vi "MIDI_JamSession_run-me.vi"() -> ()   [LabVIEW 2013]
doc: "Render a standard MIDI file to a audio using user-defined subVIs as the \"instruments\" in \"The Band.\""
uses:
  Instance           1 30Saved   MIDI_JamSession_run-me .vi
  <vilib>/Analysis/NI_AALBase.lvlib
  Instance           2 30Saved   MIDI_JamSession_run-me .vi
  Instance           3 30Saved   MIDI_JamSession_run-me .vi
  <vilib>/Analysis/baseanly.llb/Quick Scale 2D.vi
  <vilib>/Utility/file.llb/Write To Spreadsheet File (DBL).vi
panel:
  out "playing audio":bool
  in  "lock pan":bool
  in  "lock mute":bool
  in  "lock preview":bool
  in  "lock instrument":bool
  in  "preview":bool[](array[boolean])=[TRUE, TRUE, TRUE, TRUE, TRUE, TRUE, TRUE, TRUE, TRUE, TRUE, TRUE, TRUE, TRUE, TRUE, TRUE, TRUE]
  in  "random pan":bool
  in  "note events output file (.csv)":path
  out "end":string="0:00"
  out "begin":string="0:00"
  out "duration":string="0:00"
  in  "About":bool
  in  "Show help":bool
  in  "Listen":bool=TRUE
  in  "Time range to render":cluster{i32, i32}(slide)={0, 10} scale=0.0..100.0
  in  "fs [Hz]":dbl=11025.0
  in  "pan (left <==> right)":i32[](array[slide])=[0, 0, 0, 0, 0, 0, 0, 0, 0, 0, 0, 0, 0, 0, 0, 0] min=-10 max=10 scale=-10.0..10.0
  out "Audio rendering progress":u8(slide) scale=0.0..100.0
  in  "mute":bool[](array[boolean])=[FALSE, FALSE, FALSE, FALSE, FALSE, FALSE, FALSE, FALSE, FALSE, FALSE, FALSE, FALSE, FALSE, FALSE, FALSE, FALSE]
  in  "\"The Band\"":path[](array[path])=[path "", path "", path "", path "", path "", path "", path "", path "", path "", path "", path "", path "", path "", path "", path "", path ""]
  in  "audio output file (.wav)":path
  in  "Render Audio":bool
  in  "stop":bool
  out "ticks/qnote":u16
  out "tracks":u16
  out "type":u16
  out "Text":string
  out "Track number: name [channel(s) used]":string="Please select a MIDI file..."
  out "duration (min:sec)":string="0:00"
  in  "MIDI file (.mid)":path
  # "lock to channel 1"
  # "File info:"
  # "1"
  # "2"
  # "3"
  # "4"
  # "5"
  # "6"
  # "7"
  # "8"
  # "9"
  # "10"
  # "11"
  # "12"
  # "13"
  # "14"
  # "15"
  # "16"
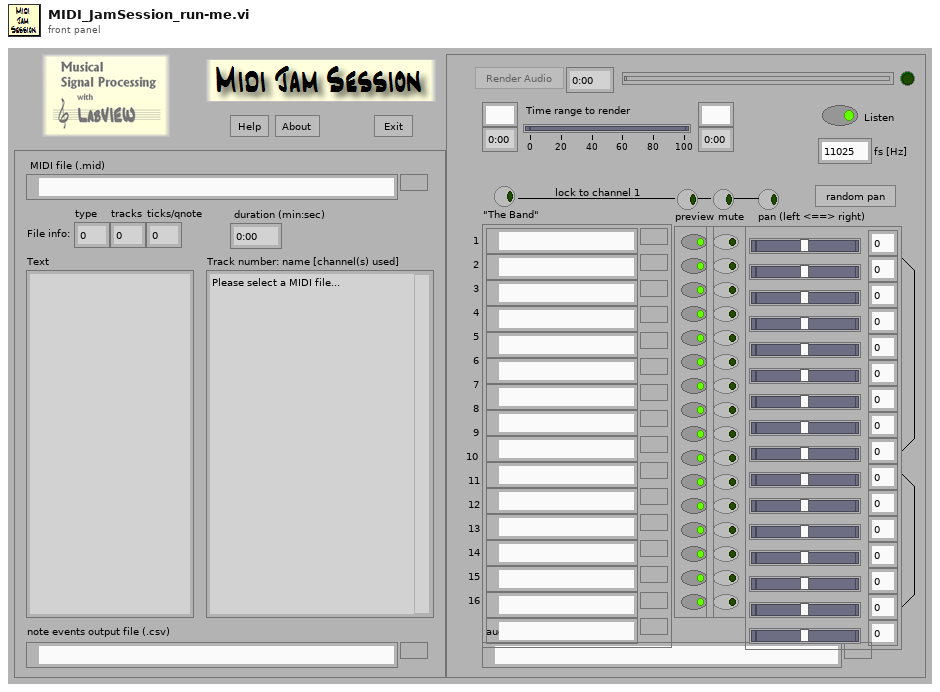
[diagram p1: front panel]
types:
  T1 = cluster{"type":u16, "tracks":u16, "ticks per qnote":u16}
  T2 = cluster{"note events":dbl[][], "duration [seconds]":dbl, "track info":string, "text meta-events":string}
  T3 = typedef "midi_NoteInfo.ctl" = cluster{"channel, 1 to 16":i32, "offset":i32, "length":i32, "frequency, 0 to 1":dbl, "amplitude, 0 to 1":dbl}
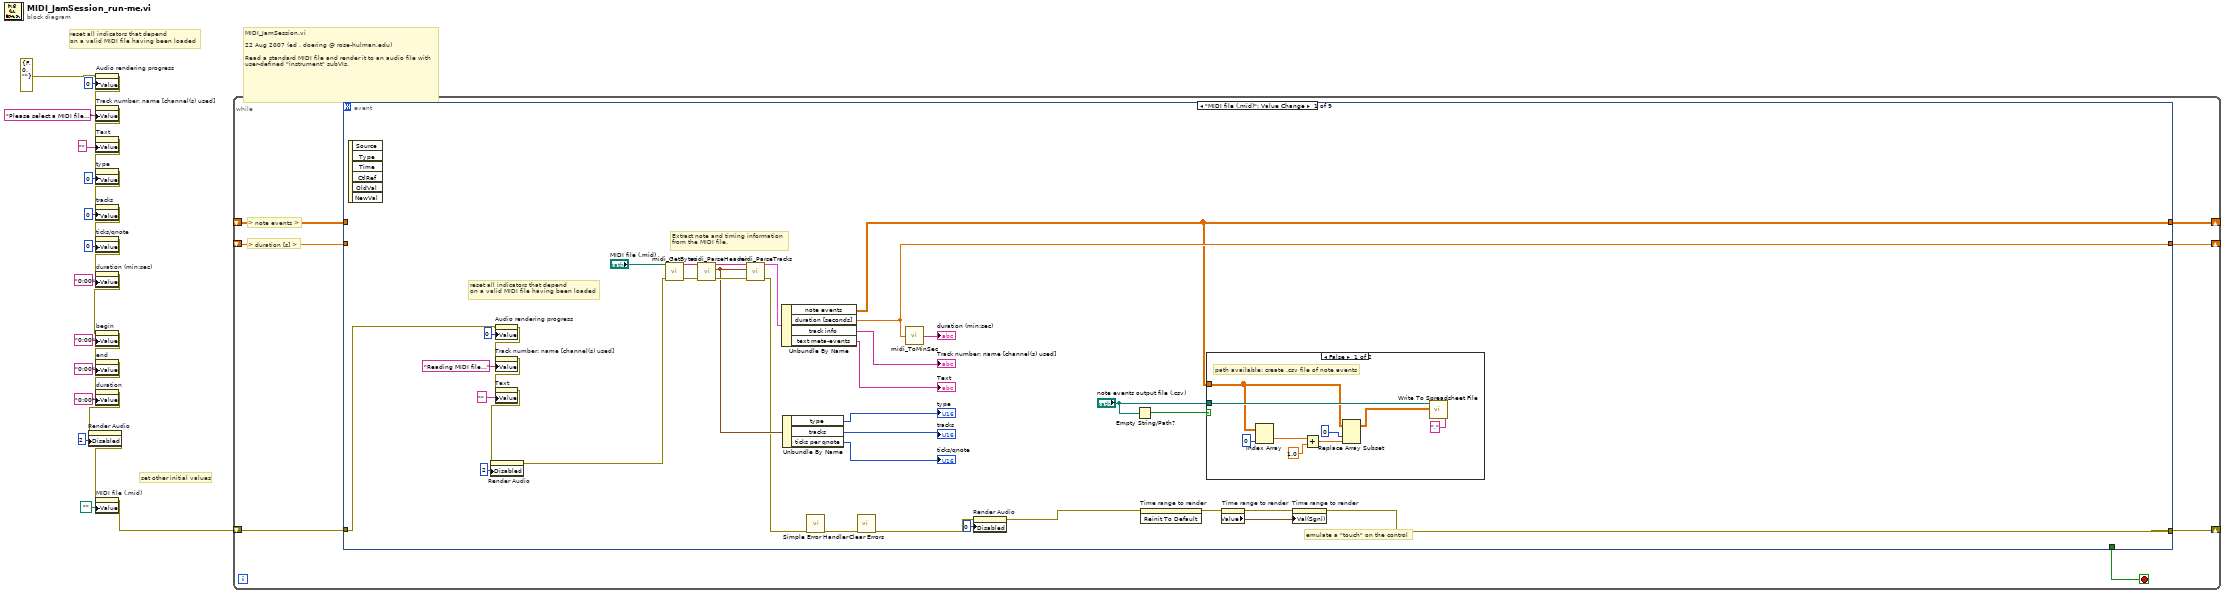
[diagram p0: block diagram]
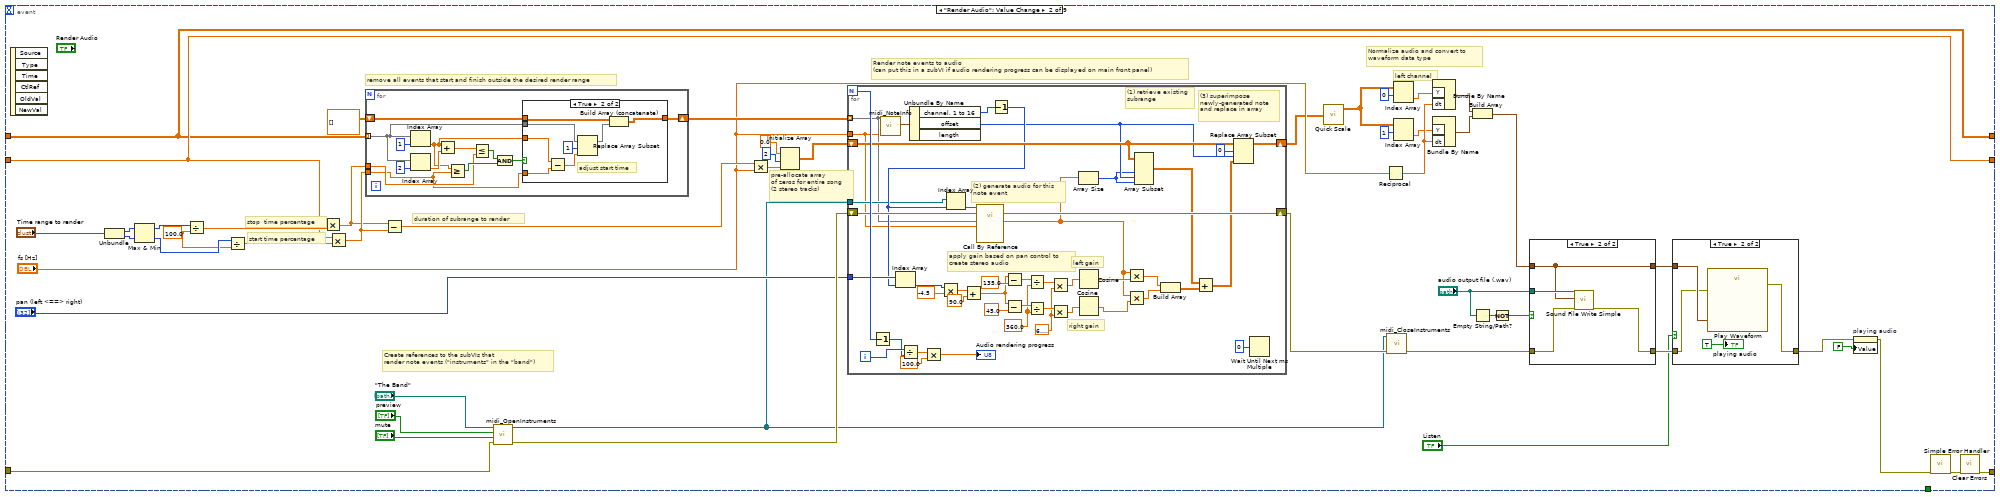
[diagram p3: hidden frame]
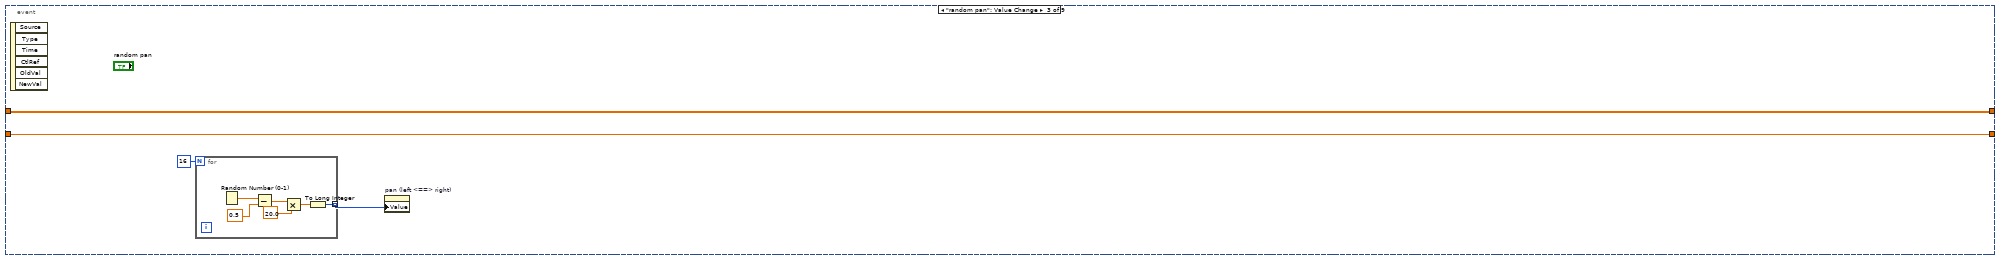
[diagram p7: hidden frame]
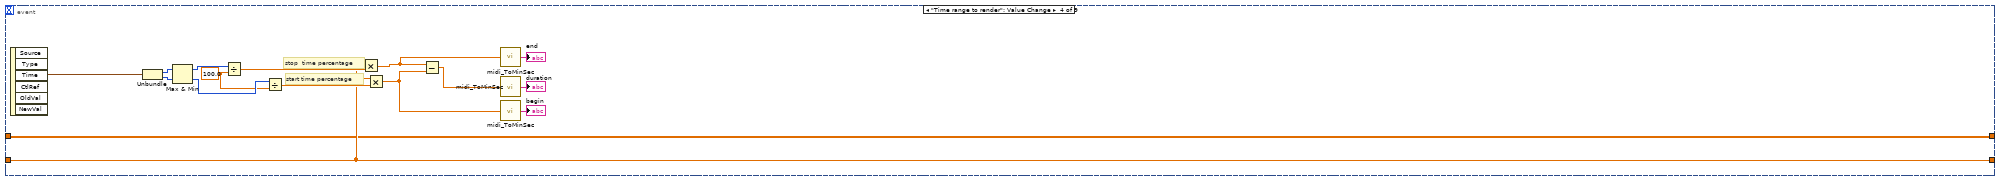
[diagram p8: hidden frame]
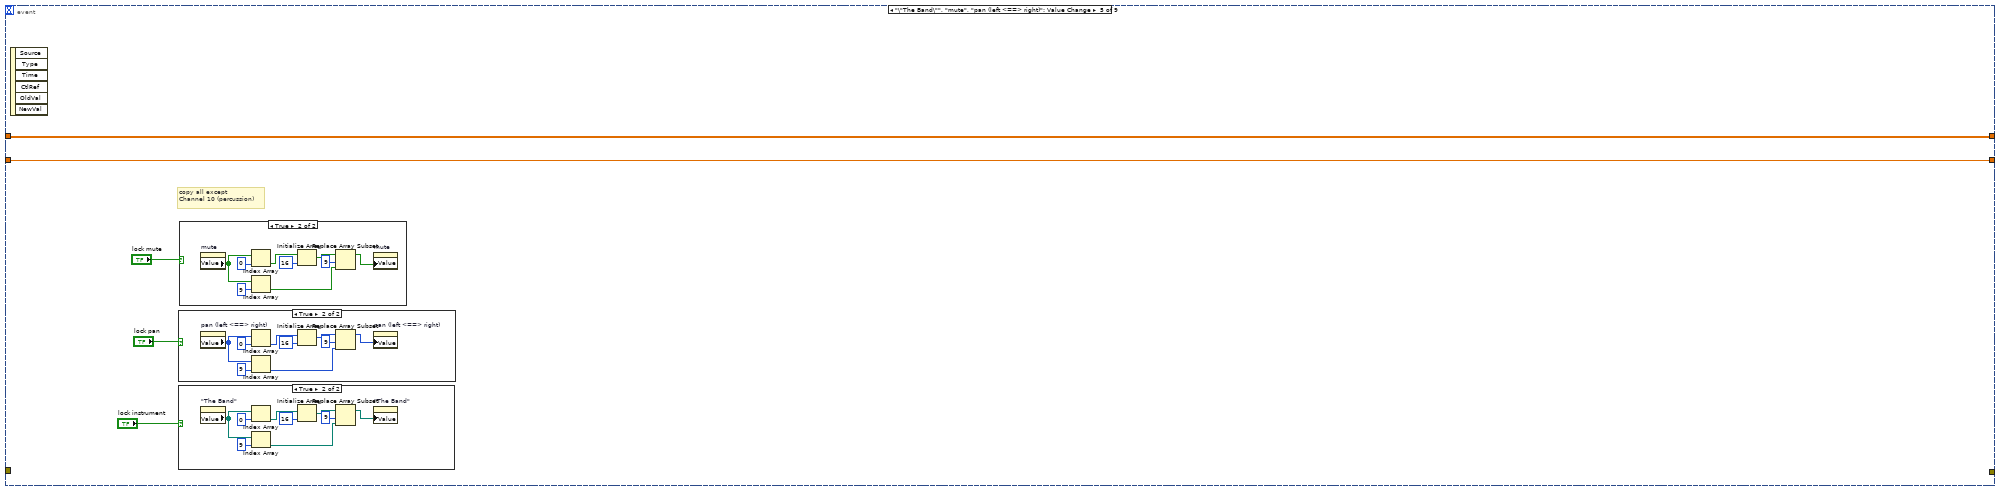
[diagram p9: hidden frame]
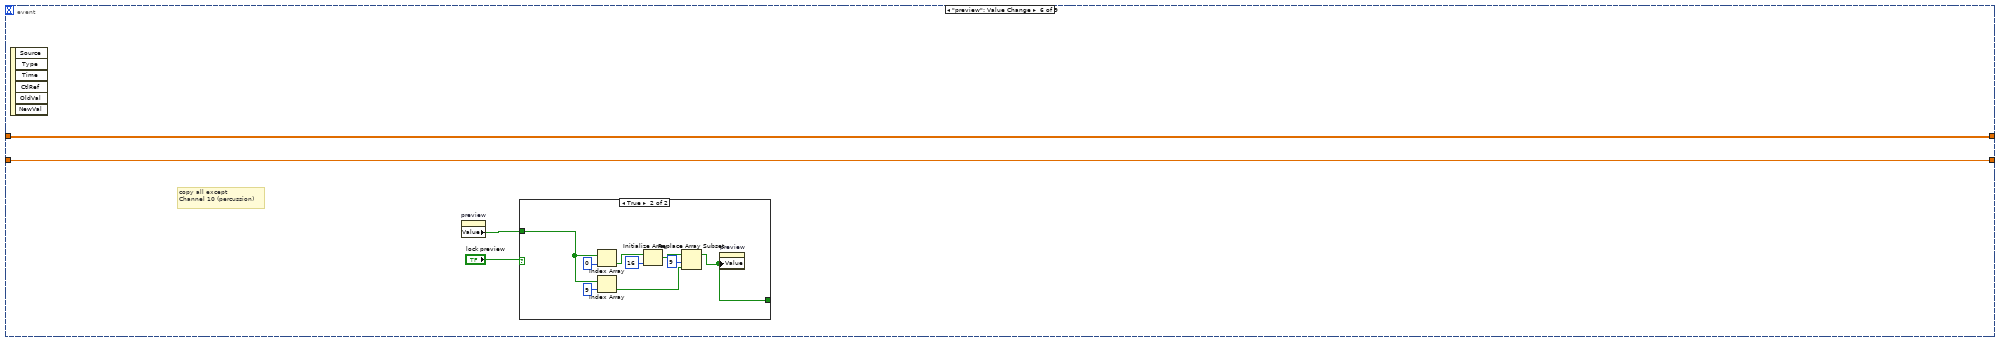
[diagram p13: hidden frame]
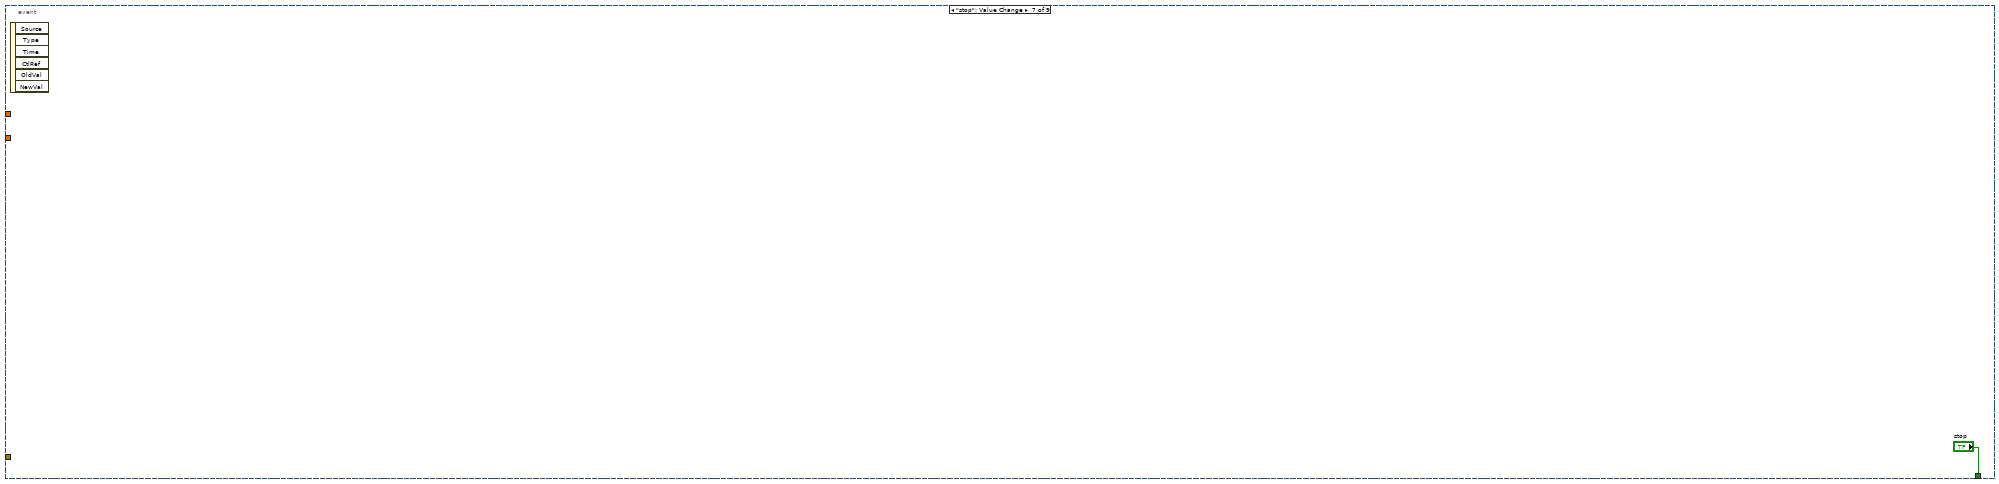
[diagram p15: hidden frame]
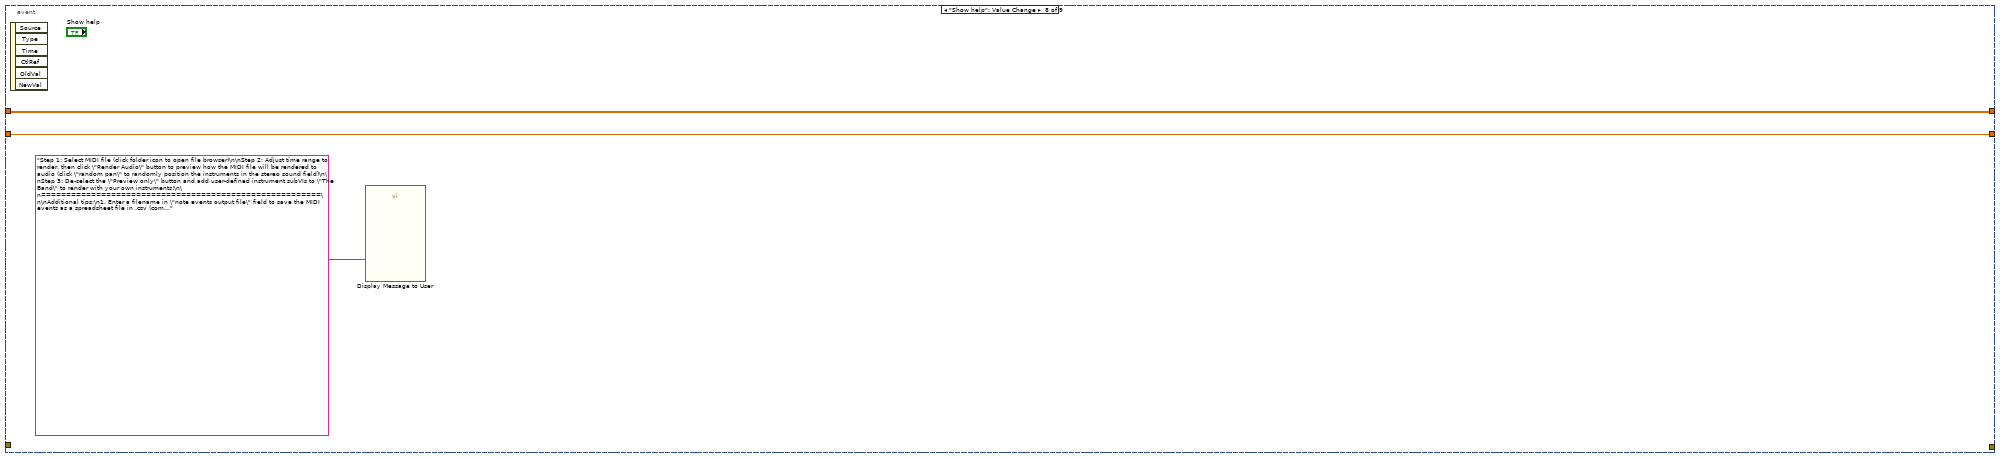
[diagram p16: hidden frame]
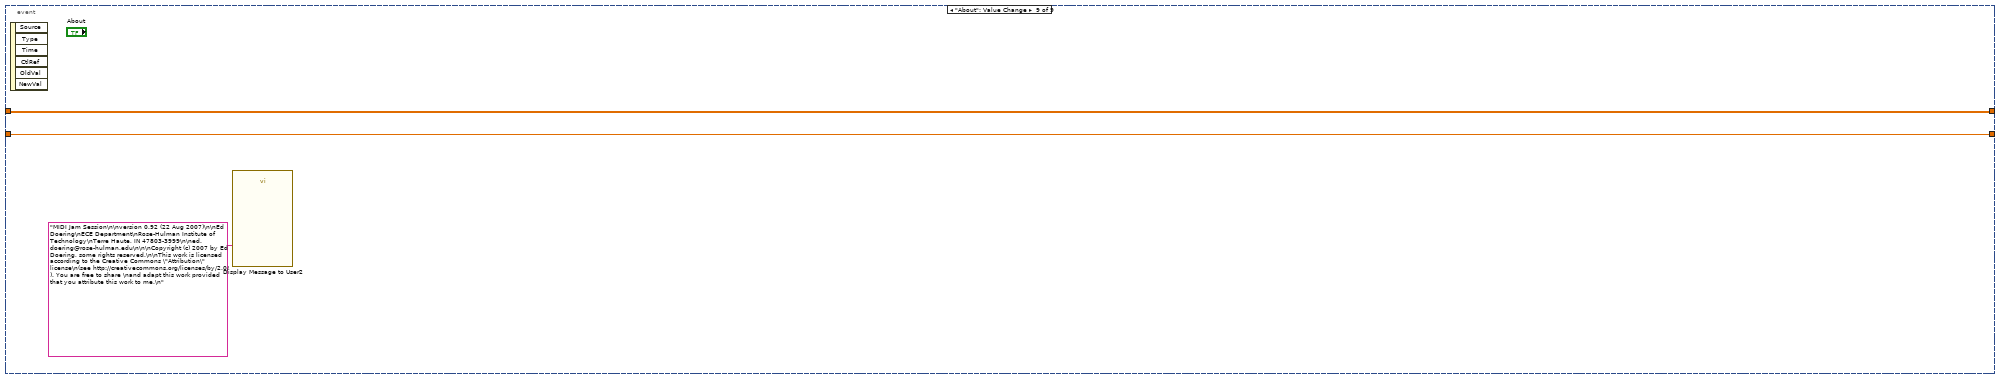
[diagram p17: hidden frame]
diagram:
  # "set other initial values"
  # "reset all indicators that depend\non a valid MIDI file having been loaded"
  # "MIDI_JamSession.vi\n\n22 Aug 2007 (ed . doering @ rose-hulman.edu)\n\nRead a standard MIDI file and render it to an audio file with\nuser-defined \"instrument\" subVIs."
  n1 = property on="Audio rendering progress" class="Slide (strict)"(error in=errorcluster {"status"=FALSE, "code"=0, "source"=""} ("error out"), "Value"=u8 0 ("Audio rendering progress")) -> (error out=w24:errorcluster)  [unwired: 1 in, 1 out]
  n2 = property on="Track number: name [channel(s) used]" class="Str"(error in=w24, "Value"="Please select a MIDI file..." ("Track number: name [channel(s) used]")) -> (error out=w25:errorcluster)  [unwired: 1 in, 1 out]
  n3 = property on="Text" class="Str"(error in=w25, "Value"="" ("Track number: name [channel(s) used]")) -> (error out=w15:errorcluster)  [unwired: 1 in, 1 out]
  n4 = property on="type" class="DigNum (strict)"(error in=w15, "Value"=u16 0 ("file type")) -> (error out=w14:errorcluster)  [unwired: 1 in, 1 out]
  n5 = property on="tracks" class="DigNum (strict)"(error in=w14, "Value"=u16 0 ("file type")) -> (error out=w13:errorcluster)  [unwired: 1 in, 1 out]
  n6 = property on="ticks/qnote" class="DigNum (strict)"(error in=w13, "Value"=u16 0 ("file type")) -> (error out=w12:errorcluster)  [unwired: 1 in, 1 out]
  n7 = property on="duration (min:sec)" class="Str"(error in=w12, "Value"="0:00" ("duration (min:sec)")) -> (error out=w2:errorcluster)  [unwired: 1 in, 1 out]
  n8 = property on="begin" class="Str"(error in=w2, "Value"="0:00" ("begin")) -> (error out=w8:errorcluster)  [unwired: 1 in, 1 out]
  n9 = property on="end" class="Str"(error in=w8, "Value"="0:00" ("begin")) -> (error out=w6:errorcluster)  [unwired: 1 in, 1 out]
  n10 = property on="duration" class="Str"(error in=w6, "Value"="0:00" ("begin")) -> (error out=w4:errorcluster)  [unwired: 1 in, 1 out]
  n11 = property on="Render Audio" class="Bool"(error in=w4, "Disabled"=u8 2) -> (error out=w3:errorcluster)  [unwired: 1 in, 1 out]
  n12 = property on="MIDI file (.mid)" class="Path"(error in=w3, "Value"=path "" ("MIDI file (.mid)")) -> (error out=w1:errorcluster)  [unwired: 1 in, 1 out]
  n13 = while {
    shift-right: [w31] -> _
    shift-left: _ -> [w28]
    shift-right: [w30] -> _
    shift-left: _ -> [w29]
    shift-right: [w27] -> _
    shift-left: w1 -> [w26]
    stop <- w32 stop-if-true
    # "> duration [s] >"
    # "> note events >"
    n14 = event shown="[0] \"MIDI file (.mid)\": Value Change" {
      selector: _ -> [_ _ _ _ _ _ _ _ _]
      dyn-events: _ -> [_ _ _ _ _ _ _ _ _]
      timeout: _ -> [_ _ _ _ _ _ _ _ _]
      tunnel: [_ _ _ _ _ _ "stop" _ _] -> w32
      tunnel: [w33 w90 w205 w215 w235 w266 _ w279 w282] -> w31
      tunnel: [w55 w91 w206 w220 w234 w265 _ w278 w281] -> w30
      tunnel: w29 -> [_ w91 w206 w220 w234 w265 _ w278 w281]
      tunnel: w28 -> [_ w90 w205 w215 w235 w266 _ w279 w282]
      tunnel: [w40 w93 _ _ _ _ _ _ _] -> w27
      tunnel: w26 -> [w46 w116 _ _ _ _ _ _ _]
      event "MIDI file (.mid)": Value Change {
        # "emulate a \"touch\" on the control"
        # "reset all indicators that depend\non a valid MIDI file having been loaded"
        # "Extract note and timing information\nfrom the MIDI file."
        n15 = event-data() -> ()  [unwired: 1 in, 6 out]
        n16 = property on="Audio rendering progress" class="Slide (strict)"(error in=w46, "Value"=u8 0 ("Audio rendering progress")) -> (error out=w48:errorcluster)  [unwired: 1 in, 1 out]
        n17 = property on="Track number: name [channel(s) used]" class="Str"(error in=w48, "Value"="Reading MIDI file..." ("Track number: name [channel(s) used]")) -> (error out=w47:errorcluster)  [unwired: 1 in, 1 out]
        n18 = property on="Text" class="Str"(error in=w47, "Value"="" ("Track number: name [channel(s) used]")) -> (error out=w37:errorcluster)  [unwired: 1 in, 1 out]
        n19 = property on="Render Audio" class="Bool"(error in=w37, "Disabled"=u8 2) -> (error out=w41:errorcluster)  [unwired: 1 in, 1 out]
        n20 = call "midi_GetBytes.vi"("error in (no error)"=w41, "folder name"="MIDI file (.mid)") -> ("error out"=w54:errorcluster, "string"=w65:string)  [unwired: 7 in, 1 out]
        n21 = call "midi_ParseHeader.vi"("error in (no error)"=w54, "string in"=w65) -> ("error out"=w63:errorcluster, "header info"=w59:T1, "string out"=w64:string)  [unwired: 7 in]
        n22 = call "midi_ParseTracks.vi"("error in (no error)"=w63, "header info"=w59, "string in"=w64) -> ("error out"=w53:errorcluster, "file contents"=w62:T2)  [unwired: 7 in]
        n23 = Unbundle By Name(w62) -> ("note events"=w33:dbl[][], "duration [seconds]"=w55:dbl, "track info"=→"Track number: name [channel(s) used]":string, "text meta-events"=→"Text":string)
        n24 = Unbundle By Name(w59) -> ("type"=→"type":u16, "tracks"=→"tracks":u16, "ticks per qnote"=→"ticks/qnote":u16)
        n25 = call <vilib>:"Simple Error Handler.vi"("error in (no error)"=w53) -> ("error out"=w52:errorcluster)  [unwired: 4 in, 4 out]
        n26 = call <vilib>:"Clear Errors.vi"("error in (no error)"=w52) -> ("error out"=w38:errorcluster)  [unwired: 6 in]
        n27 = call "midi_ToMinSec.vi"("seconds"=w55) -> ("min:sec"=→"duration (min:sec)":string)
        n28 = property on="Render Audio" class="Bool"(error in=w38, "Disabled"=u8 0) -> (error out=w36:errorcluster)  [unwired: 1 in, 1 out]
        n29 = Empty String/Path?(string/path="note events output file (.csv)") -> (empty?=w35:bool)
        n30 = invoke on="Time range to render" class="Slide (strict)" method="Reinit To Default"(error in=w36) -> (error out=w43:errorcluster)  [unwired: 2 in, 2 out]
        n31 = case shown="False" w35 {
          tunnel: "note events output file (.csv)" -> [w75 _]
          tunnel: w33 -> [w71 _]
          frame False {
            # "path available: create .csv file of note events"
            n32 = Index Array(array=w71, index (col)=0 ("disabled index (col)")) -> (element=w72:dbl[])  [unwired: 1 in]
            n33 = Add(x=w72, y=1.0) -> (x+y=w69:dbl[])
            n34 = Replace Array Subset(array=w71, new element=w69, index (col)=0 ("disabled index (col)")) -> (w68:dbl[][])  [unwired: 1 in]
            n35 = call-poly <vilib>:"Write To Spreadsheet File.vi"("delimiter (\\t)"="," ("delimiter (\\t)"), "2D data"=w68, "file path (dialog if empty)"=w75) -> ()  [unwired: 5 in, 1 out]
          }
          frame True {
            # "path empty: do not create .csv file"
          }
        }
        n36 = property on="Time range to render" class="Slide (strict)"(error in=w43) -> (error out=w45:errorcluster, "Value"=w44:cluster{i32, i32})  [unwired: 1 in, 1 out]
        n37 = property on="Time range to render" class="Slide (strict)"(error in=w45, "Val(Sgnl)"=w44) -> (error out=w40:errorcluster)  [unwired: 1 in, 1 out]
      }
      event "Render Audio": Value Change {
        w117 = 100.0 ("y")
        # "left channel"
        # "Normalize audio and convert to\nwaveform data type"
        # "Render note events to audio\n(can put this in a subVI if audio rendering progress can be displayed on main front panel)"
        # "pre-allocate array\nof zeros for entire song\n(2 stereo tracks)"
        # "duration of subrange to render"
        # "Create references to the subVIs that\nrender note events (\"instruments\" in the \"band\")"
        # "start time percentage"
        # "stop  time percentage"
        # "remove all events that start and finish outside the desired render range"
        n38 = event-data() -> ()  [unwired: 1 in, 6 out]
        n39 = Unbundle("Time range to render") -> (w119:i32, w120:i32)
        n40 = Max & Min(x=w119, y=w120) -> (max(x,y)=w124:i32, min(x,y)=w121:i32)
        n41 = Divide(x=w124, y=w117) -> (x/y=w122:dbl)
        n42 = Divide(x=w121, y=w117) -> (x/y=w123:dbl)
        n43 = Multiply(x=w91, y=w122) -> (x*y=w125:dbl)
        n44 = Multiply(x=w91, y=w123) -> (x*y=w126:dbl)
        n45 = for {
          tunnel: w90 -> [w193] mode=indexing
          tunnel: w125 -> [w185]
          shift-right: [w192] -> w110
          shift-left: dbl[][] [] -> [w191]
          tunnel: w126 -> [w184]
          n46 = Index Array(array=w193, index=1) -> (element=w183:dbl)
          n47 = Index Array(array=w193, index=2) -> (element=w190:dbl)
          n48 = Add(x=w183, y=w190) -> (x+y=w189:dbl)
          n49 = Greater Or Equal?(x=w183, y=w184) -> (x >= y?=w187:bool)
          n50 = Less Or Equal?(x=w189, y=w185) -> (x <= y?=w188:bool)
          n51 = And(x=w188, y=w187) -> (x .and. y?=w186:bool)
          n52 = case shown="True" w186 {
            tunnel: w193 -> [_ w202]
            tunnel: [w196 w204] -> w192
            tunnel: w191 -> [w196 w203]
            tunnel: w183 -> [_ w200]
            tunnel: w184 -> [_ w199]
            frame False {
            }
            frame True {
              # "adjust start time"
              n53 = Subtract(x=w200, y=w199) -> (x-y=w198:dbl)
              n54 = Replace Array Subset(array=w202, new element=w198, index=1) -> (w197:dbl[])
              n55 = Build Array (concatenate)(w203, w197) -> (w204:dbl[][])
            }
          }
        }
        n56 = Subtract(x=w125, y=w126) -> (x-y=w111:dbl)
        n57 = call "midi_OpenInstruments.vi"("error in (no error)"=w116, "mute"="mute", "preview"="preview", "instruments"="\"The Band\"") -> ("error out"=w101:errorcluster, "vi references"=w95:refnum<vi>[])  [unwired: 6 in]
        n58 = Multiply(x=w111, y="fs [Hz]") -> (x*y=w114:dbl)
        n59 = Initialize Array(0.0 ("element"), 2 ("dimension size"), w114) -> (w112:dbl[][])
        n60 = for {
          N -> [w178]
          shift-right: [w163] -> w86
          shift-left: w112 -> [w161]
          shift-right: [w177] -> w100
          shift-left: w101 -> [w175]
          tunnel: "pan (left <==> right)" -> [w174]
          tunnel: w110 -> [w153] mode=indexing
          tunnel: "fs [Hz]" -> [w152]
          tunnel: w95 -> [w155]
          i -> [w181]
          w149 = 360.0 ("y")
          w146 = 6.283185307179586
          # "apply gain based on pan control to\ncreate stereo audio"
          # "right gain"
          # "left gain"
          # "(2) generate audio for this\nnote event"
          # "(3) superimpose\nnewly-generated note\nand replace in array"
          # "(1) retrieve existing\nsubrange"
          n61 = Decrement(x=w178) -> (x-1=w179:i32)
          n62 = call "midi_NoteInfo.vi"("fs [Hz]"=w152, "note event"=w153) -> ("note info"=w159:T3)  [unwired: 9 in]
          n63 = Divide(x=w181, y=w179) -> (x/y=w182:dbl)
          n64 = Unbundle By Name(w159) -> ("channel, 1 to 16"=w158:i32, "offset"=w157:i32)  [unwired: 1 out]
          n65 = Multiply(x=w182, y=100.0) -> (x*y=→"Audio rendering progress":dbl)
          n66 = Decrement(x=w158) -> (x-1=w160:i32)
          n67 = Index Array(array=w174, index=w160) -> (element=w170:i32)
          n68 = Multiply(x=w170, y=-4.5) -> (x*y=w172:dbl)
          n69 = Index Array(array=w155, index=w160) -> (element=w176:refnum<vi>)
          n70 = Add(x=w172, y=90.0) -> (x+y=w167:dbl)
          n71 = call-by-ref "?"(reference=w176, error in=w175, "fs (Hz)"=w152, "note"=w153) -> (error out=w177:errorcluster, "audio"=w139:dbl[])  [unwired: 9 in, 1 out]
          n72 = Subtract(x=w167, y=135.0) -> (x-y=w151:dbl)
          n73 = Subtract(x=w167, y=45.0) -> (x-y=w150:dbl)
          n74 = Divide(x=w151, y=w149) -> (x/y=w148:dbl)
          n75 = Divide(x=w150, y=w149) -> (x/y=w147:dbl)
          n76 = Multiply(x=w148, y=w146) -> (x*y=w144:dbl)
          n77 = Multiply(x=w147, y=w146) -> (x*y=w145:dbl)
          n78 = Array Size(array=w139) -> (size(s)=w138:i32)
          n79 = Cosine(x=w144) -> (cos(x)=w143:dbl)
          n80 = Cosine(x=w145) -> (cos(x)=w142:dbl)
          n81 = Multiply(x=w139, y=w143) -> (x*y=w140:dbl[])
          n82 = Multiply(x=w139, y=w142) -> (x*y=w141:dbl[])
          n83 = Array Subset(array=w161, length (row)=w138, index (col)=w157, length (col)=w138) -> (w165:dbl[][])  [unwired: 1 in]
          n84 = Build Array(w140, w141) -> (w166:dbl[][])
          n85 = Add(x=w165, y=w166) -> (x+y=w164:dbl[][])
          n86 = Replace Array Subset(array=w161, new element=w164, index (row)=0 ("disabled index (col)"), index (col)=w157) -> (w163:dbl[][])
          n87 = Wait Until Next ms Multiple(millisecond multiple=u32 0) -> ()  [unwired: 1 out]
        }
        n88 = call-poly <vilib>:"Quick Scale.vi"("X"=w86) -> ("Yij=Xij/Max|X|"=w85:dbl[][])  [unwired: 2 out]
        n89 = Reciprocal(x="fs [Hz]") -> (1/x=w106:dbl)
        n90 = call "midi_CloseInstruments.vi"("error in (no error)"=w100, "vi references"=w95) -> ("error out"=w103:errorcluster)  [unwired: 9 in]
        n91 = Index Array(array=w85, index (row)=0 ("index")) -> (element=w87:dbl[])  [unwired: 1 in]
        n92 = Index Array(array=w85, index (row)=1 ("index")) -> (element=w88:dbl[])  [unwired: 1 in]
        n93 = Bundle By Name("Y"=w87, "dt"=w106) -> (w109:waveform(dbl))  [unwired: 1 in]
        n94 = Bundle By Name("Y"=w88, "dt"=w106) -> (w105:waveform(dbl))  [unwired: 1 in]
        n95 = Build Array(w109, w105) -> (w89:waveform(dbl)[])
        n96 = Empty String/Path?(string/path="audio output file (.wav)") -> (empty?=w84:bool)
        n97 = Not(x=w84) -> (.not. x?=w82:bool)
        n98 = case shown="True" w82 {
          tunnel: [w128 w131] -> w104
          tunnel: "audio output file (.wav)" -> [_ w132]
          tunnel: w89 -> [w127 w129]
          tunnel: w103 -> [w128 w130]
          tunnel: [w127 w129] -> w102
          frame False {
          }
          frame True {
            n99 = call <vilib>:"Sound File Write Simple.vi"("error in (no error)"=w130, "data"=w129, "path"=w132) -> ("error out"=w131:errorcluster)  [unwired: 7 in, 1 out]
          }
        }
        n100 = case shown="True" "Listen" {
          tunnel: w102 -> [_ w137]
          tunnel: [w133 w136] -> w79
          tunnel: w104 -> [w133 w135]
          frame False {
          }
          frame True {
            n101 = call "Play Waveform"("Data"=w137, "error in"=w135) -> ("error out"=w136:errorcluster)  [unwired: 17 in]
            "playing audio" <- TRUE ("playing audio")
          }
        }
        n102 = property on="playing audio" class="Bool (strict)"(error in=w79, "Value"=FALSE ("playing audio")) -> (error out=w78:errorcluster)  [unwired: 1 in, 1 out]
        n103 = call <vilib>:"Simple Error Handler.vi"("error in (no error)"=w78) -> ("error out"=w94:errorcluster)  [unwired: 4 in, 4 out]
        n104 = call <vilib>:"Clear Errors.vi"("error in (no error)"=w94) -> ("error out"=w93:errorcluster)  [unwired: 6 in]
      }
      event "random pan": Value Change {
        n105 = event-data() -> ()  [unwired: 1 in, 6 out]
        n106 = for {
          N: 16 -> [_]
          tunnel: [w209] -> w207 mode=indexing
          n107 = Random Number (0-1)() -> (number: 0 to 1=w213:dbl)
          n108 = Subtract(x=w213, y=0.5) -> (x-y=w211:dbl)
          n109 = Multiply(x=w211, y=20.0) -> (x*y=w210:dbl)
          n110 = To Long Integer(number=w210) -> (32bit integer=w209:i32)
        }
        n111 = property on="pan (left <==> right)" class="Arr (strict)"("Value"=w207) -> ()  [unwired: 2 in, 2 out]
      }
      event "Time range to render": Value Change {
        w224 = 100.0 ("y")
        # "start time percentage"
        # "stop  time percentage"
        n112 = event-data() -> ("NewVal"=w223:cluster{i32, i32})  [unwired: 1 in, 5 out]
        n113 = Unbundle(w223) -> (w225:i32, w226:i32)
        n114 = Max & Min(x=w225, y=w226) -> (max(x,y)=w230:i32, min(x,y)=w227:i32)
        n115 = Divide(x=w230, y=w224) -> (x/y=w228:dbl)
        n116 = Divide(x=w227, y=w224) -> (x/y=w229:dbl)
        n117 = Multiply(x=w220, y=w228) -> (x*y=w216:dbl)
        n118 = Multiply(x=w220, y=w229) -> (x*y=w218:dbl)
        n119 = Subtract(x=w216, y=w218) -> (x-y=w222:dbl)
        n120 = call "midi_ToMinSec.vi"("seconds"=w216) -> ("min:sec"=→"end":string)
        n121 = call "midi_ToMinSec.vi"("seconds"=w222) -> ("min:sec"=→"duration":string)
        n122 = call "midi_ToMinSec.vi"("seconds"=w218) -> ("min:sec"=→"begin":string)
      }
      event "\"The Band\"", "mute", "pan (left <==> right)": Value Change {
        # "copy all except\nChannel 10 (percussion)"
        n123 = event-data() -> ()  [unwired: 1 in, 6 out]
        n124 = case shown="True" "lock pan" {
          frame False {
          }
          frame True {
            n125 = property on="pan (left <==> right)" class="Arr (strict)"() -> ("Value"=w246:i32[])  [unwired: 2 in, 2 out]
            n126 = Index Array(array=w246, index=0) -> (element=w249:i32)
            n127 = Index Array(array=w246, index=9) -> (element=w253:i32)
            n128 = Initialize Array(w249, 16 ("dimension size")) -> (w250:i32[])
            n129 = Replace Array Subset(array=w250, new element=w253, index=9) -> (w245:i32[])
            n130 = property on="pan (left <==> right)" class="Arr (strict)"("Value"=w245) -> ()  [unwired: 2 in, 2 out]
          }
        }
        n131 = case shown="True" "lock instrument" {
          frame False {
          }
          frame True {
            n132 = property on="\"The Band\"" class="Arr (strict)"() -> ("Value"=w239:path[])  [unwired: 2 in, 2 out]
            n133 = Index Array(array=w239, index=0) -> (element=w242:path)
            n134 = Index Array(array=w239, index=9) -> (element=w237:path)
            n135 = Initialize Array(w242, 16 ("dimension size")) -> (w241:path[])
            n136 = Replace Array Subset(array=w241, new element=w237, index=9) -> (w236:path[])
            n137 = property on="\"The Band\"" class="Arr (strict)"("Value"=w236) -> ()  [unwired: 2 in, 2 out]
          }
        }
        n138 = case shown="True" "lock mute" {
          frame False {
          }
          frame True {
            n139 = property on="mute" class="Arr (strict)"() -> ("Value"=w255:bool[])  [unwired: 2 in, 2 out]
            n140 = Index Array(array=w255, index=0) -> (element=w258:bool)
            n141 = Index Array(array=w255, index=9) -> (element=w262:bool)
            n142 = Initialize Array(w258, 16 ("dimension size")) -> (w259:bool[])
            n143 = Replace Array Subset(array=w259, new element=w262, index=9) -> (w254:bool[])
            n144 = property on="mute" class="Arr (strict)"("Value"=w254) -> ()  [unwired: 2 in, 2 out]
          }
        }
      }
      event "preview": Value Change {
        # "copy all except\nChannel 10 (percussion)"
        n145 = event-data() -> ()  [unwired: 1 in, 6 out]
        n146 = property on="preview" class="Arr (strict)"() -> ("Value"=w264:bool[])  [unwired: 2 in, 2 out]
        n147 = case shown="True" "lock preview" {
          tunnel: [w267 w269] -> _
          tunnel: w264 -> [w267 w268]
          frame False {
          }
          frame True {
            n148 = Index Array(array=w268, index=0) -> (element=w274:bool)
            n149 = Index Array(array=w268, index=9) -> (element=w270:bool)
            n150 = Initialize Array(w274, 16 ("dimension size")) -> (w273:bool[])
            n151 = Replace Array Subset(array=w273, new element=w270, index=9) -> (w269:bool[])
            n152 = property on="preview" class="Arr (strict)"("Value"=w269) -> ()  [unwired: 2 in, 2 out]
          }
        }
      }
      event "stop": Value Change {
        n153 = event-data() -> ()  [unwired: 1 in, 6 out]
      }
      event "Show help": Value Change {
        n154 = event-data() -> ()  [unwired: 1 in, 6 out]
        n155 = call "Display Message to User"("Message"="Step 1: Select MIDI file (click folder icon to open file browser)\n\nStep 2: Adjust time range to render, then click \"Render Audio\" button to preview how the MIDI file will be rendered to audio (click \"random pan\" to randomly position the instruments in the stereo sound field)\n\nStep 3: De-select the \"Preview only\" button and add user-defined instrument subVIs to \"The Band\" to render with your own instruments!\n\n========================================================\n\nAdditional tips:\n1. Enter a filename in \"note events output file\" field to save the MIDI events as a spreadsheet file in .csv (comma-separated values) format; the file will be created immediately after the MIDI file is loaded. The columns are: channel number (1 to 16), start time (in seconds), duration (in seconds), note number (0 to 127), and velocity (0 to 127).\n\n2. Enter a filename in \"audio output file\" to save rendered audio to a .wav file; the file will be created new each time you press the \"Render Audio\" button.\n\n3. Select a \"lock to 1\" button to make the channel controls  track the values selected for Channel 1 (except Channel 10, percussion). This provides a quick way to mute or unmute all channels, for example.\n\n4. Blank entries in \"The Band\" will render as muted when the \"Preview only\" button is de-selected.\n\n5. De-select \"Listen\" for long pieces, since there is no way to interrupt the built-in audio player.\n\n6. See the \"readme_instructions.txt\" file in the .zip distribution for more detailed instructions!     ") -> ()  [unwired: 9 in, 2 out]
      }
      event "About": Value Change {
        n156 = event-data() -> ()  [unwired: 1 in, 6 out]
        n157 = call "Display Message to User2"("Message"="MIDI Jam Session\n\nversion 0.92 (22 Aug 2007)\n\nEd Doering\nECE Department\nRose-Hulman Institute of Technology\nTerre Haute, IN 47803-3999\n\ned.doering@rose-hulman.edu\n\n\nCopyright (c) 2007 by Ed Doering, some rights reserved.\n\nThis work is licensed according to the Creative Commons \"Attribution\" license\n(see http://creativecommons.org/licenses/by/2.0/). You are free to share \nand adapt this work provided that you attribute this work to me.\n") -> ()  [unwired: 9 in, 2 out]
      }
    }
  }
